vi "Log Results.vi"(8 "error in (no error)":errorcluster, 10 "Result":refnum<class "Mag Lab Result.lvclass">, 11 "Cap Bank Server in":refnum<class "Cap Bank Server.lvclass">) -> (0 "error out":errorcluster, 3 "Cap Bank Server out":refnum<class "Cap Bank Server.lvclass">)   [LabVIEW 2015, in "Cap Bank Server.lvclass"]
uses:
  Cap Bank Server.lvclass
  Mag Lab Result/Mag Lab Result.lvclass
  Cap Bank Server.lvclass/Cap Bank Server.ctl
  File/Controls/File formats.ctl
  <vilib>/ActorFramework/Actor/Actor.lvclass/Actor.ctl
  <vilib>/ActorFramework/Message Enqueuer/Message Enqueuer.lvclass/Message Enqueuer.ctl
  Mag Lab Measure Controller Messages/Log Status Update Msg/Log Status Update Msg.lvclass/Log Status Update Msg.ctl
  <vilib>/ActorFramework/Message Enqueuer/Init from Existing Queue.vi
  <vilib>/ActorFramework/Message Enqueuer/Enqueue.vi
  <vilib>/ActorFramework/Message Priority Queue/Priority Enqueue.vi
  <vilib>/ActorFramework/Message Enqueuer/Message Enqueuer.lvclass
  Mag Lab Measure Controller Messages/Log Status Update Msg/Log Status Update Msg.lvclass
  <vilib>/ActorFramework/Actor/Actor.lvclass
  Mag Lab Error Handler/Mag Lab Error Handler.lvclass
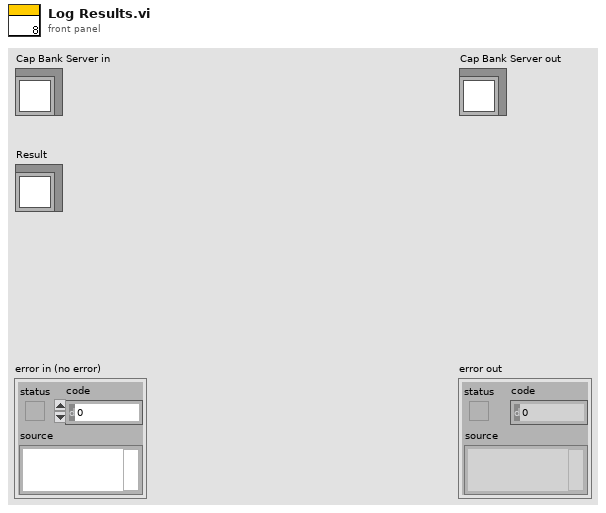
[diagram p1: front panel]
types:
  T1 = enum16{"open", "open or create", "create or replace", "create", "open (read-only)"}
  T2 = typedef "File formats.ctl" = enum16{"TDMS", "ASCII", "BINARY"}
  T3 = typedef "Shot data.ctl" = cluster{"Shot number":i32, "Time":timestamp, "Magnet ID":string, "User":string, "Cell number":i32, "Requested field":dbl, "Field direction":string, "Number of bank frames":i32, "Crowbar resistance, mOhm":dbl, "Magnet resistance, mOhm":dbl, "Charger voltage, kV":dbl, "Frame voltage, kV":dbl}
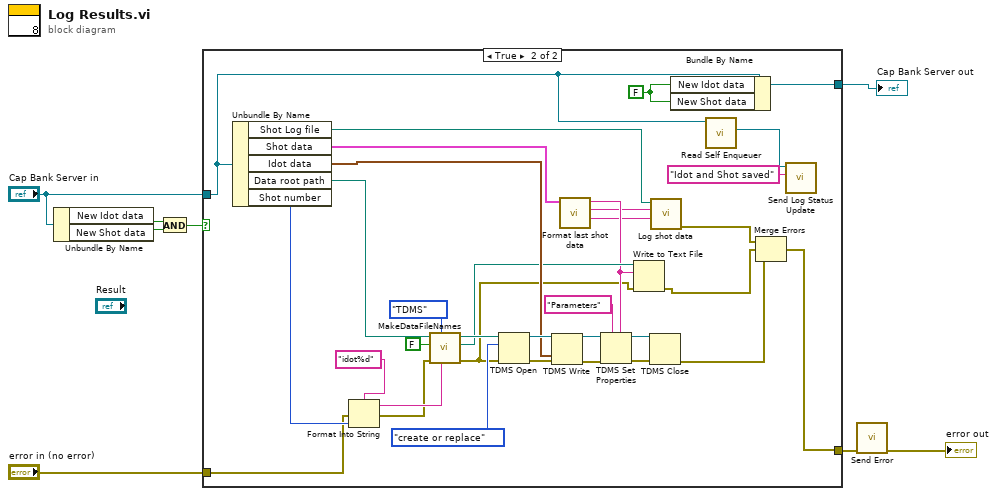
[diagram p0: block diagram]
diagram:
  n1 = Unbundle By Name("Cap Bank Server in") -> ("New Idot data"=w7:bool, "New Shot data"=w8:bool)
  n2 = And(x=w7, y=w8) -> (x .and. y?=w6:bool)
  n3 = case shown="True" w6 {
    tunnel: "Cap Bank Server in" -> [w10 w12]
    tunnel: [w10 w44] -> w4
    tunnel: [w9 w16] -> w3
    tunnel: "error in (no error)" -> [w9 w14]
    frame False {
    }
    frame True {
      w43 = FALSE ("New Idot data")
      n4 = Unbundle By Name(w12) -> ("Shot Log file"=w20:path, "Shot data"=w28:T3, "Idot data"=w32:waveform(dbl)[], "Data root path"=w41:path, "Shot number"=w39:i32)
      n5 = Format Into String(format string="idot%d", error in=w14, w39) -> (resulting string=w38:string, error out=w15:errorcluster)  [unwired: 1 in]
      n6 = call "MakeDataFileNames.vi"("File Prefix"=w38, "File format"=File_formats."TDMS", "Error In"=w15, "Generate Index"=FALSE, "Root Data Folder"=w41) -> ("Error Out"=w23:errorcluster, "Settings File Path"=w25:path, "Data File  Path"=w36:path)  [unwired: 3 in, 1 out]
      n7 = TDMS Open(8:w23, 10:T1."create or replace" ("operation (0:open)"), 11:w36) -> (0:w33:errorcluster, 3:w34:refnum<k34>)  [unwired: 4 in]
      n8 = TDMS Write(0:w34, 9:w32, 11:w33) -> (4:w30:refnum<k34>, 15:w31:errorcluster)  [unwired: 3 in, 2 out]
      n9 = call "Format last shot data.vi"("Shot data"=w28) -> ("Spreadsheet header string"=w21:string, "Spreadsheet shot string"=w22:string, "Formated shot data"=w24:string)  [unwired: 6 in, 2 out]
      n10 = TDMS Set Properties(5:w24, 7:"Parameters", 8:w31, 11:w30) -> (0:w27:errorcluster, 3:w26:refnum<k34>)  [unwired: 2 in, 2 out]
      n11 = Write to Text File(file (use dialog)=w25, text=w24, error in=w23) -> (error out=w18:errorcluster)  [unwired: 1 in, 2 out]
      n12 = TDMS Close(8:w27, 11:w26) -> (0:w17:errorcluster)  [unwired: 1 out]
      n13 = call "Log shot data.vi"("Spreadsheet header string"=w21, "Spreadsheet shot string"=w22, "Log file folder"=w20) -> ("error out"=w19:errorcluster)  [unwired: 7 in, 1 out]
      n14 = Bundle By Name(cluster=w12, "New Idot data"=w43, "New Shot data"=w43) -> (w44:refnum<class "Cap Bank Server.lvclass">)
      n15 = call <vilib>:"Read Self Enqueuer.vi"("Actor"=w12) -> ("Self Enqueuer"=w11:refnum<class "Message Enqueuer.lvclass">)  [unwired: 10 in]
      n16 = Merge Errors(w19, w18, w17) -> (w16:errorcluster)
      n17 = call "Send Log Status Update.vi"("Status"="Idot and Shot saved", "Message Enqueuer"=w11) -> ()  [unwired: 8 in, 2 out]
    }
  }
  "Cap Bank Server out" <- w4
  n18 = call "Send Error.vi"("error in (no error)"=w3) -> ("error out"=→"error out":errorcluster)  [unwired: 9 in, 1 out]
